vi "CreateSentencesFromStrings.vi"(8 "error in":errorcluster, 10 "String 2":string="BDV = 500 V.", 11 "String 1":string) -> (0 "error out":errorcluster, 3 "String 1. String 2":string)   [LabVIEW 2018]
doc: "Concatenates two strings by creating a sentence from each of them. The first letter of each string is converted to upper case. Each string is terminated by \".\" if there is no \".,? or !\" already present at the end of the string. The sentences are separated by space."
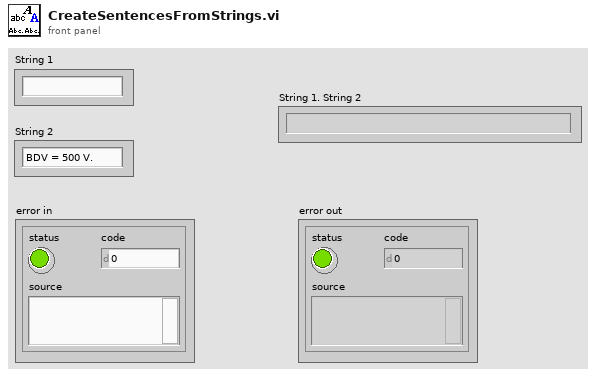
[diagram p1: front panel]
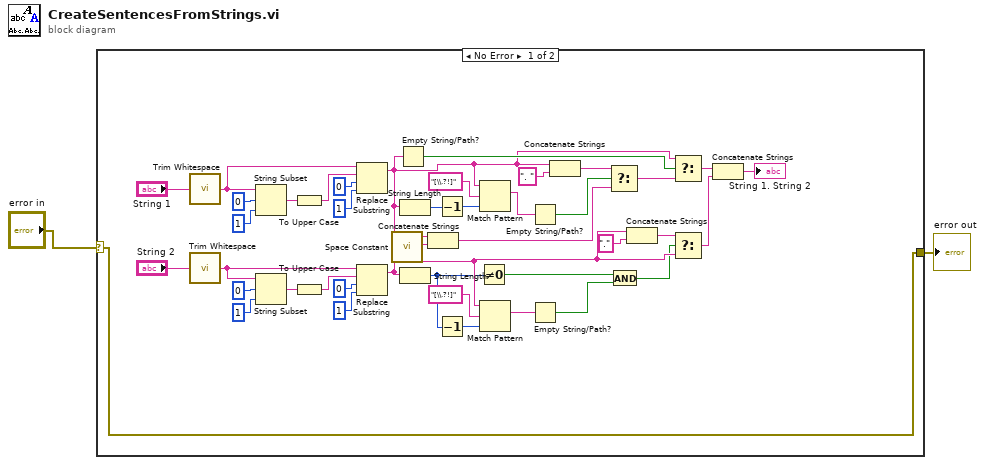
[diagram p0: block diagram]
diagram:
  n1 = case shown="No Error" "error in" {
    selector: "error in" -> [w3 w45]
    tunnel: [w3 w45] -> w1
    frame No Error {
      n2 = call <vilib>:"Trim Whitespace.vi"("string"="String 1") -> ("trimmed string"=w20:string)  [unwired: 1 in]
      n3 = call <vilib>:"Trim Whitespace.vi"("string"="String 2") -> ("trimmed string"=w9:string)  [unwired: 1 in]
      n4 = String Subset(string=w20, offset (0)=0, length (rest)=1 ("length (rest)")) -> (substring=w21:string)
      n5 = String Subset(string=w9, offset (0)=0, length (rest)=1 ("length (rest)")) -> (substring=w13:string)
      n6 = To Upper Case(1:w21) -> (0:w19:string)
      n7 = To Upper Case(1:w13) -> (0:w12:string)
      n8 = Replace Substring(2:1 ("length (len. of substring)"), 3:0 ("offset (0)"), 4:w19, 5:w20) -> (1:w16:string)  [unwired: 1 out]
      n9 = Replace Substring(2:1 ("length (len. of substring)"), 3:0 ("offset (0)"), 4:w12, 5:w9) -> (1:w8:string)  [unwired: 1 out]
      n10 = call <vilib>:"Space Constant.vi"() -> ("String"=w35:string)
      n11 = Empty String/Path?(string/path=w16) -> (empty?=w41:bool)
      n12 = String Length(string=w16) -> (length=w44:i32)
      n13 = String Length(string=w8) -> (length=w4:i32)
      n14 = Concatenate Strings(w16, w35) -> (w34:string)
      n15 = Decrement(x=w44) -> (x-1=w43:i32)
      n16 = Decrement(x=w4) -> (x-1=w29:i32)
      n17 = Not Equal To 0?(x=w4) -> (x != 0?=w7:bool)
      n18 = Match Pattern(string=w16, regular expression="[\\.?!]", offset (0)=w43) -> (match substring=w40:string)  [unwired: 3 out]
      n19 = Match Pattern(string=w8, regular expression="[\\.?!]", offset (0)=w29) -> (match substring=w27:string)  [unwired: 3 out]
      n20 = Empty String/Path?(string/path=w40) -> (empty?=w39:bool)
      n21 = Empty String/Path?(string/path=w27) -> (empty?=w6:bool)
      n22 = Concatenate Strings(w16, ". ") -> (w37:string)
      n23 = Select(t=w37, s=w39, f=w34) -> (s? t:f=w33:string)
      n24 = And(x=w7, y=w6) -> (x .and. y?=w5:bool)
      n25 = Concatenate Strings(w8, "." ("string")) -> (w25:string)
      n26 = Select(t=w16, s=w41, f=w33) -> (s? t:f=w32:string)
      n27 = Select(t=w25, s=w5, f=w8) -> (s? t:f=w24:string)
      n28 = Concatenate Strings(w32, w24) -> (→"String 1. String 2":string)
    }
    frame Error {
    }
  }
  "error out" <- w1
